vi "Write Arm Position Values.vi"(8 "error in (no error)":errorcluster, 10 "Arm Positions":T1, 11 "Elevator in":refnum<class "Elevator.lvclass">) -> (0 "error out":errorcluster, 3 "Elevator out":refnum<class "Elevator.lvclass">)   [LabVIEW 2019, in "Elevator.lvlib" / "Elevator.lvclass"]
uses:
  Elevator.lvclass
  Controls/Arm Position Values.ctl
  Elevator.lvclass/Elevator.ctl
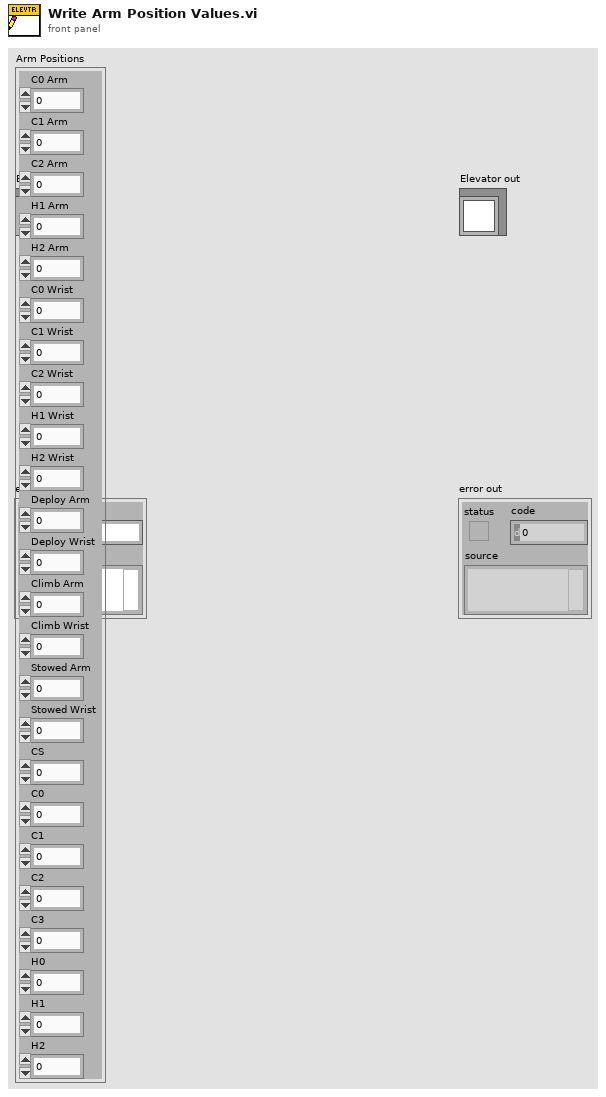
[diagram p1: front panel]
types:
  T1 = typedef "Elevator.lvlib/Elevator.lvclass/Arm Position Values.ctl" = cluster{"C0 Arm":dbl, "C1 Arm":dbl, "C2 Arm":dbl, "H1 Arm":dbl, "H2 Arm":dbl, "C0 Wrist":dbl, "C1 Wrist ":dbl, "C2 Wrist":dbl, "H1 Wrist":dbl, "H2 Wrist":dbl, "Deploy Arm":dbl, "Deploy Wrist":dbl, "Climb Arm":dbl, "Climb Wrist":dbl, "Stowed Arm":dbl, "Stowed Wrist":dbl, "CS":dbl, "C0":dbl, "C1":dbl, "C2":dbl, "C3":dbl, "H0":dbl, "H1":dbl, "H2":dbl}
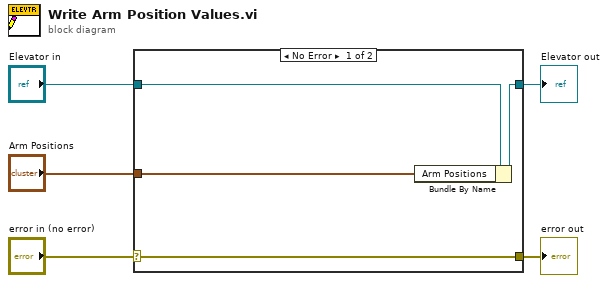
[diagram p0: block diagram]
diagram:
  n1 = case shown="No Error" "error in (no error)" {
    selector: "error in (no error)" -> [w9 w10]
    tunnel: [w9 w10] -> w4
    tunnel: [w7 w11] -> w2
    tunnel: "Elevator in" -> [w8 w11]
    tunnel: "Arm Positions" -> [w6 _]
    frame No Error {
      n2 = Bundle By Name(cluster=w8, "Arm Positions"=w6) -> (w7:refnum<class "Elevator.lvclass">)
    }
    frame Error {
    }
  }
  "error out" <- w4
  "Elevator out" <- w2
